vi "ITX to HDF5.vi"(8 "error in (no error)":errorcluster, 11 "file (use dialog)":path=path "C:/") -> (0 "error out":errorcluster)   [LabVIEW 2019, in "Conversion.lvclass"]
uses:
  Conversion.lvclass
  Data/Data.lvclass
  Data/Typedefs/File Type--enum.ctl
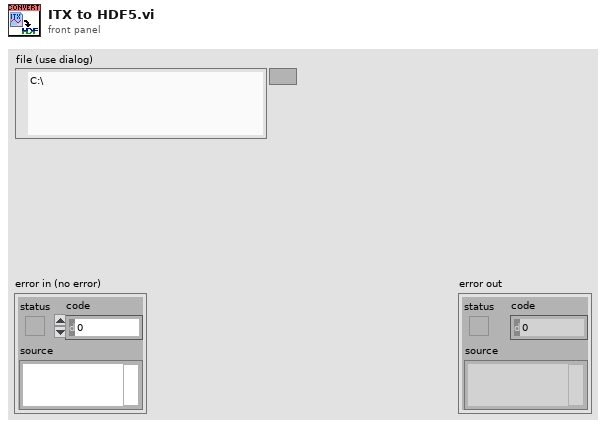
[diagram p1: front panel]
types:
  T1 = typedef "Data.lvclass/File Type--enum.ctl" = enum16{"DAT", "ITX", "HDF5", "TDMS", "VI", "PGSQL"}
  T2 = typedef "Data.lvclass/Dictionary--cluster.ctl" = cluster{"key":string, "value":variant}
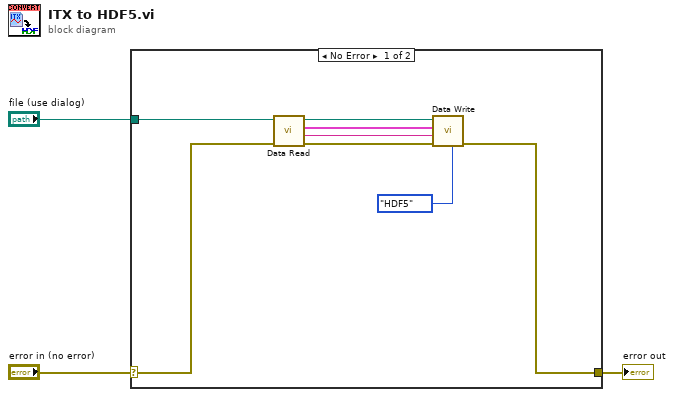
[diagram p0: block diagram]
diagram:
  n1 = case shown="No Error" "error in (no error)" {
    selector: "error in (no error)" -> [w6 w12]
    tunnel: [w5 w12] -> w2
    tunnel: "file (use dialog)" -> [w11 _]
    frame No Error {
      n2 = call "Data Read.vi"("error in (no error)"=w6, "path"=w11) -> ("error out"=w9:errorcluster, "Notes"=w8:string, "Data (Dictionary)"=w7:T2[], "path out"=w10:path)  [unwired: 6 in]
      n3 = call "Data Write.vi"("File Type"=File_Type--enum."HDF5", "error in (no error)"=w9, "Notes"=w8, "Data (Dictionary)"=w7, "path"=w10) -> ("error out"=w5:errorcluster)  [unwired: 5 in, 1 out]
    }
    frame Error {
    }
  }
  "error out" <- w2
